vi "Agitator Loop.vi"() -> ()   [LabVIEW 2016]
uses:
  Robot Global Data.vi
  Common Code/Shooter Commands.ctl
panel:
  out "Spread your wings and learn how to fly?":bool
  out "Intake Power":dbl
  out "Stir Power":dbl
  out "Override Everything?":bool
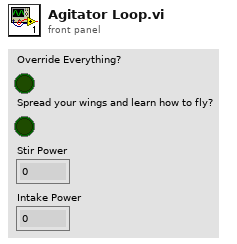
[diagram p1: front panel]
types:
  T1 = typedef "Shooter Commands.ctl" = enum16{"Idle ", "Warmup ", "Shoot"}
  T2 = typedef "Dashboard Control Data.ctl" = cluster{"Drivetrain Settings":T3, "Intake Presets ":T5, "Shooter Presets":T6, "Vision Target Packet":T7, "Auton Presets":cluster{"Start Position":dbl}, "Drivetrain Encoder Values":T8, "Drivetrain Encoder Settings":cluster{"Left Tick Constant":dbl, "Right Tick Contant":dbl, "Reset Encoders":bool, "Center Tick Constant":dbl}, "Zero Gyro":bool, "Vision Timeout":dbl, "Pressure M":dbl, "Pressure B":dbl, "Auto Agitator":T10}
  T3 = typedef "Drivetrain Settings.ctl" = cluster{"Gyro Tolerance":dbl, "Gyro Steer PID Gains":T4, "Y Power Multiplier":dbl, "Turn Power Multiplier":dbl, "Gyro Output":dbl, "Creep Rate":dbl, "Distance Drive PID Gains":T4, "Distance Tolerance":dbl, "Distance Output":dbl, "Strafe Threshold":dbl, "Strafe Correct":bool, "Strafe Corect Tolerance":dbl, "Translate Drive PID Gains":T4, "Strafe Output":dbl, "SC Right":dbl, "SC Left":dbl, "Use Gyro":bool, "Constant Power":bool, "Strafe Power":dbl}
  T4 = typedef "PID Gains.ctl" = cluster{"proportional gain (Kc)":dbl, "integral time (Ti, min)":dbl, "derivative time (Td, min)":dbl}
  T5 = typedef "Intake Presets.ctl" = cluster{"Intake Speed ":dbl, "Outake Speed":dbl, "Current Trip Delay":dbl, "Max Current":dbl}
  T6 = typedef "Shooter Presets.ctl" = cluster{"Key Shot":cluster{"RPM ":dbl, "Hood?":bool}, "Distance Shot":cluster{"RPM":dbl, "Hood?":bool}, "RPM Tolerance":dbl, "Unstuck Delay Time ":dbl, "Initial RPM Increase":dbl, "Warmup Delay":dbl, "Faster Time":dbl, "Shooter PID Gains":cluster{"P":dbl, "I":dbl, "D":dbl, "FF":dbl, "Ramp Rate":dbl, "I Zone":dbl}, "Unstuck Trigger Power":dbl, "Trigger Power":dbl, "Unstuck RPM":dbl, "Agitator Active Power":dbl, "Agitator Idle Power":dbl}
  T7 = typedef "Vision Target Packet.ctl" = cluster{"Robot Center":dbl, "Center X":dbl, "Center Y":dbl, "Angle":dbl, "Distance":dbl, "Found Target?":bool}
  T8 = typedef "Drivetrain Encoder Values.ctl" = cluster{"Left Encoder":T9, "Center Encoder":T9, "Right Encoder":T9}
  T9 = typedef "Encoder Values.ctl" = cluster{"Distance":dbl, "Speed":dbl, "Tick":dbl}
  T10 = typedef "Auto Agitator Settings.ctl" = cluster{"Enable Auto Agitation":bool, "Continuous Stir":bool, "Continuous Intake":bool, "Alternate In/Outtake":bool, "Wing Delay":dbl, "Stir Delay":dbl, "Intake Delay":dbl, "Wing On Time":dbl, "Wing Off Time":dbl, "Stir On Time":dbl, "Stir Off Time":dbl, "Intake On Time":dbl, "Intake Off Time":dbl, "Stir Power":dbl, "Intake Power":dbl, "Outtake Power":dbl, "Intake Run Time":dbl, "Outtake Run Time":dbl, "Wing$":bool, "Intake":bool, "Stirrer":bool}
  T11 = typedef "Shooter Status Cluster.ctl" = cluster{"Current RPM":dbl, "Trigger Power":dbl, "Shooter Mode":T12, "Shot Type":T13, "Shooter State":T1, "Target RPM":dbl, "Hood Down?":bool, "RPM Reached?":bool}
  T12 = typedef "Shooter Modes.ctl" = enum16{"Auto", "Manual"}
  T13 = typedef "Shot Type.ctl" = enum16{"Vision Shot", "Dist Shot", "Key Shot"}
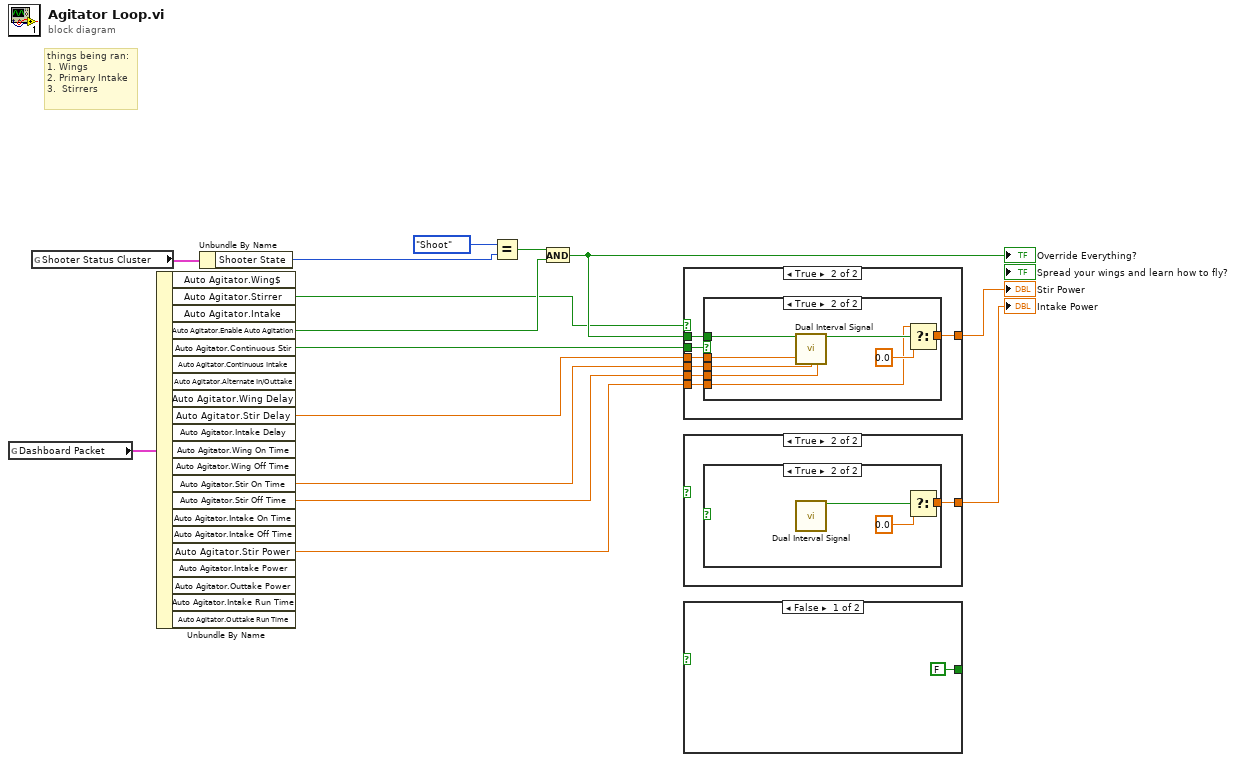
[diagram p0: block diagram]
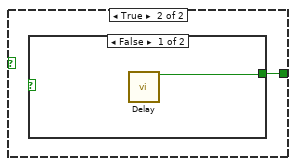
[diagram p2: hidden frame]
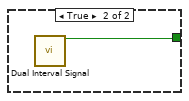
[diagram p3: hidden frame]
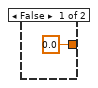
[diagram p4: hidden frame]
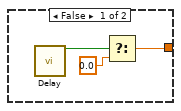
[diagram p5: hidden frame]
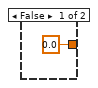
[diagram p6: hidden frame]
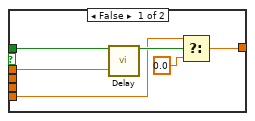
[diagram p7: hidden frame]
diagram:
  # "things being ran:\n1. Wings\n2. Primary Intake\n3.  Stirrers"
  n1 = global read "Robot Global Data.vi" "Dashboard Packet"() -> (w10:T2)
  n2 = global read "Robot Global Data.vi" "Shooter Status Cluster"() -> (w15:T11)
  n3 = Unbundle By Name(w10) -> ("Auto Agitator.Stirrer"=w3:bool, "Auto Agitator.Enable Auto Agitation"=w9:bool, "Auto Agitator.Continuous Stir"=w2:bool, "Auto Agitator.Stir Delay"=w8:dbl, "Auto Agitator.Stir On Time"=w7:dbl, "Auto Agitator.Stir Off Time"=w6:dbl, "Auto Agitator.Stir Power"=w5:dbl)  [unwired: 14 out]
  n4 = Unbundle By Name(w15) -> ("Shooter State"=w14:T1)
  n5 = Equal?(x=Shooter_Commands."Shoot" ("Shooter State"), y=w14) -> (x = y?=w12:bool)
  n6 = And(x=w12, y=w9) -> (x .and. y?=w4:bool)
  "Override Everything?" <- w4
  n7 = case shown="True" w3 {
    tunnel: [0.0 ("f") w23] -> w11
    tunnel: w8 -> [_ w21]
    tunnel: w7 -> [_ w20]
    tunnel: w6 -> [_ w19]
    tunnel: w5 -> [_ w18]
    tunnel: w4 -> [_ w22]
    tunnel: w2 -> [_ w17]
    frame False {
    }
    frame True {
      n8 = case shown="True" w17 {
        tunnel: [w26 w36] -> w23
        tunnel: w22 -> [w29 w35]
        tunnel: w21 -> [w28 w33]
        tunnel: w20 -> [_ w32]
        tunnel: w19 -> [_ w31]
        tunnel: w18 -> [w24 w30]
        frame False {
          n9 = call "Delay.vi"("Enable?"=w29, "Delay"=w28) -> ("Output"=w27:bool)  [unwired: 13 in]
          n10 = Select(t=w24, s=w27, f=0.0) -> (s? t:f=w26:dbl)
        }
        frame True {
          n11 = call "Dual Interval Signal.vi"("Enable?"=w35, "Delay"=w33, "On Time"=w32, "Off Time"=w31) -> ("Output"=w34:bool)  [unwired: 11 in]
          n12 = Select(t=w30, s=w34, f=0.0) -> (s? t:f=w36:dbl)
        }
      }
    }
  }
  "Stir Power" <- w11
  n13 = case shown="True" {
    selector: _ -> [_ _]
    tunnel: [0.0 ("f") w39] -> w1
    frame False {
    }
    frame True {
      n14 = case shown="True" {
        selector: _ -> [_ _]
        tunnel: [w41 w44] -> w39
        frame False {
          n15 = call "Delay.vi"() -> ("Output"=w42:bool)  [unwired: 15 in]
          n16 = Select(s=w42, f=0.0) -> (s? t:f=w41:dbl)  [unwired: 1 in]
        }
        frame True {
          n17 = call "Dual Interval Signal.vi"() -> ("Output"=w43:bool)  [unwired: 15 in]
          n18 = Select(s=w43, f=0.0) -> (s? t:f=w44:dbl)  [unwired: 1 in]
        }
      }
    }
  }
  "Intake Power" <- w1
  n19 = case shown="False" {
    selector: _ -> [_ _]
    tunnel: [FALSE ("Output") w47] -> _
    frame False {
    }
    frame True {
      n20 = case shown="False" {
        selector: _ -> [_ _]
        tunnel: [w48 w49] -> w47
        frame False {
          n21 = call "Delay.vi"() -> ("Output"=w48:bool)  [unwired: 15 in]
        }
        frame True {
          n22 = call "Dual Interval Signal.vi"() -> ("Output"=w49:bool)  [unwired: 15 in]
        }
      }
    }
  }
